vi "Set-Exit.vi"(8 "error in (no error)":errorcluster, 10 "Exit?":bool, 11 "UI ref. in":refnum<data-value>) -> (0 "error out":errorcluster, 3 "UI ref.":refnum<data-value>)   [LabVIEW 2013, in "CameraVision.lvlib" / "CV-UI.lvclass"]
uses:
  CV-UI.lvclass
  CV-UI.lvclass/CV-UI.ctl
  Read Exit.vi
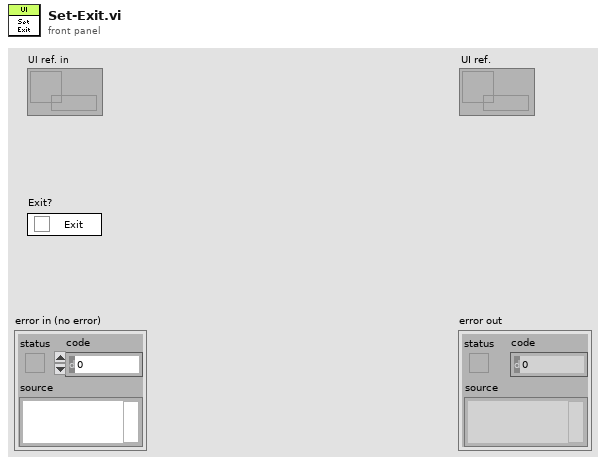
[diagram p1: front panel]
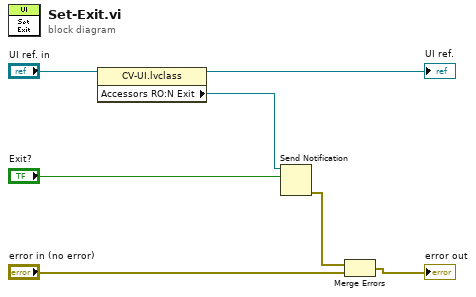
[diagram p0: block diagram]
diagram:
  n1 = property class="CV-UI.lvclass"(reference="UI ref. in") -> (reference out=→"UI ref.":refnum<data-value>, "Accessors RO:N Exit"=w3:refnum<notifier>)  [unwired: 1 in, 1 out]
  n2 = Send Notification(notification="Exit?", notifier=w3) -> (error out=w7:errorcluster)  [unwired: 1 in, 1 out]
  n3 = Merge Errors(w7, "error in (no error)") -> (→"error out":errorcluster)
